vi "Error Handler.vi"(9 "Ignore Errors":i32[](array[numeric]), 10 "error to process":errorcluster, 11 "Message Queue":T1) -> (2 "Enqueued Error?":bool, 3 "Message Queue dub":T1)   [LabVIEW 2019, in "Test.lvlib"]
doc: "Check the 'error to process' to see if its code value matches any of the values in the 'Ignore Errors' array. If so, do nothing. If not, send an \"Error\" message containing the error data to the Message Handling Loop for further processing."
uses:
  Test.lvlib
  Support/Shared/TypeDefs/Message Queue Ref.ctl
  Message Queue/State Name.ctl
  Message Queue/Enqueue (Single).vi
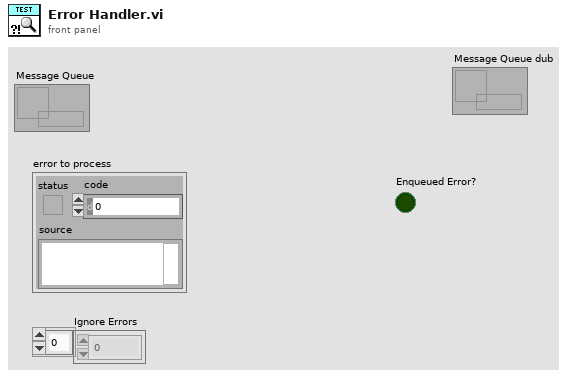
[diagram p1: front panel]
types:
  T1 = typedef "Message Queue Ref.ctl" = refnum<queue>
  T2 = typedef "Test.lvlib/State Name.ctl" = enum16{"Default", "Initialize", "Re-Initialize", "Initialize Data", "Initialize Panel", "[Event Structure] Update Data", "Error", "Exit"}
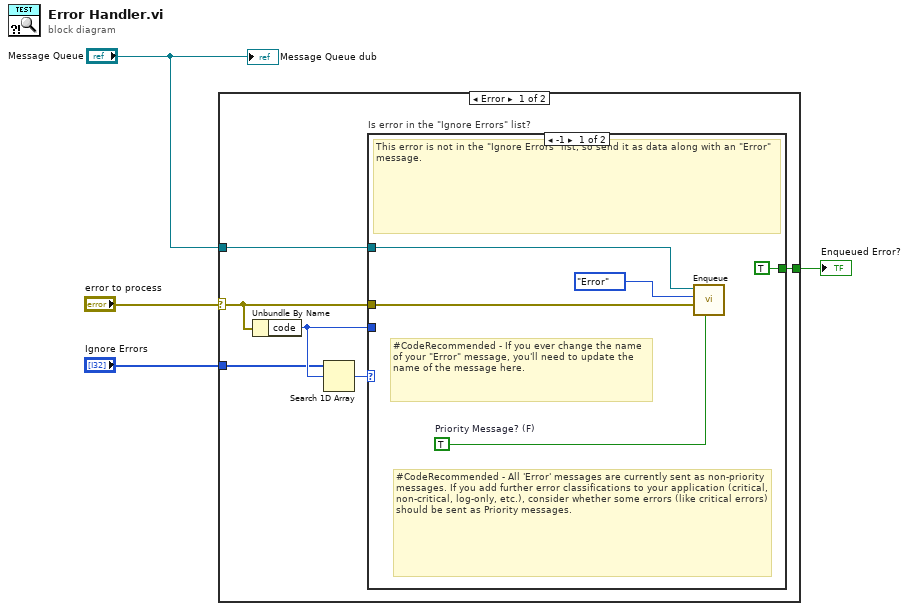
[diagram p0: block diagram]
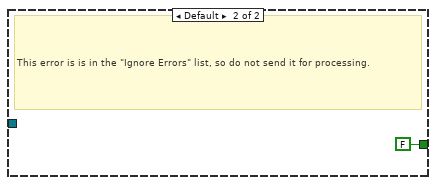
[diagram p2: hidden frame]
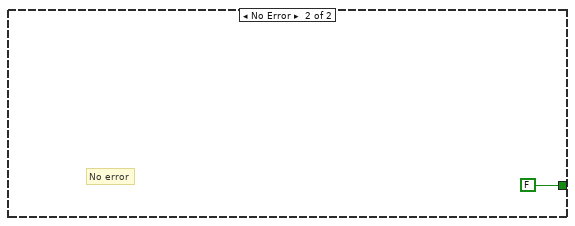
[diagram p3: hidden frame]
diagram:
  n1 = case shown="Error" "error to process" {
    selector: "error to process" -> [w7 _]
    tunnel: "Message Queue" -> [w10 _]
    tunnel: "Ignore Errors" -> [w6 _]
    tunnel: [w5 FALSE] -> w2
    frame Error {
      n2 = Unbundle By Name(w7) -> ("code"=w8:i32)
      n3 = Search 1D Array(1D array=w6, element=w8) -> (index of element=w9:i32)  [unwired: 1 in]
      n4 = case "Is error in the \"Ignore Errors\" list?" shown="-1" w9 {
        tunnel: w7 -> [w12 _]
        tunnel: w10 -> [w14 _]
        tunnel: w8 -> [_ _]
        tunnel: [TRUE FALSE] -> w5
        frame -1 {
          w11 = TRUE  # Priority Message? (F)
          # "#CodeRecommended - All 'Error' messages are currently sent as non-priority messages. If you add further error classifications to your application (critical, non-critical, log-only, etc.), consider whether some errors (like critical errors) should be sent as Priority messages."
          # "#CodeRecommended - If you ever change the name of your \"Error\" message, you'll need to update the name of the message here."
          # "This error is not in the \"Ignore Errors\" list, so send it as data along with an \"Error\" message."
          n5 = call-poly "Enqueue.vi"("Priority Message? Array"=w11, "Message Data Array"=w12, "States"=State_Name."Error" ("Array"), "Message Queue"=w14) -> ()  [unwired: 6 in, 2 out]
        }
        frame Default {
          # "This error is is in the \"Ignore Errors\" list, so do not send it for processing."
        }
      }
    }
    frame No Error {
      # "No error"
    }
  }
  "Enqueued Error?" <- w2
  "Message Queue dub" <- "Message Queue"
